vi "fpga_setup.vi"(8 "error in":errorcluster) -> (0 "error out":errorcluster, 3 "Cluster":cluster{"FPGA VI Reference Out":T1})   [LabVIEW 2014]
uses:
  fpga_reference.ctl
  <vilib>/userdefined/High Color/nirio_resource_hc.ctl
  <vilib>/FPGAPlugInAG/PCIe-7842R/niLvFpga_Open_PCIe-7842R.vi
  <vilib>/FPGAPlugInAG/PCIe-7842R/niLvFpga_Reset_PCIe-7842R.vi
  <vilib>/rvi/interface/nirviOpenFPGA/nirviOpenFPGA.xnode
  FPGA Bitfiles/i2cmuxdemux.lvbitx
  <vilib>/rvi/interface/nirviMethod/nirviMethod.xnode
panel:
  # "Open FPGA I2C interface, creating FPGA reference handle, and reset, but don't actually\nstart the hardware yet.  This will stop the hardware if it is already running."
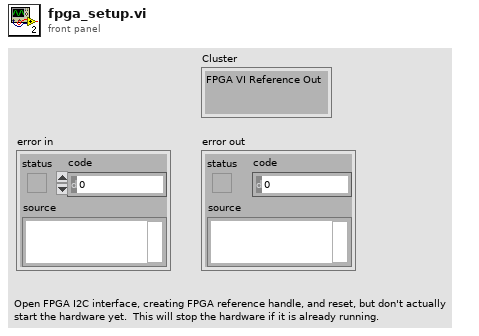
[diagram p1: front panel]
types:
  T1 = typedef "fpga_reference.ctl" = refnum<k20>
  T2 = typedef "nirio_resource_hc.ctl" = tag
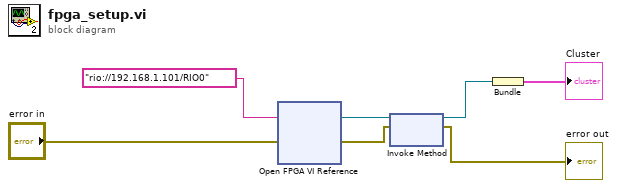
[diagram p0: block diagram]
diagram:
  n1 = xnode "Open FPGA VI Reference"("error in"="error in", "resource name"=T2 "rio://192.168.1.101/RIO0") -> ("FPGA VI Reference Out"=w5:T1, "error out"=w4:errorcluster)
  n2 = xnode "Invoke Method"("FPGA VI Reference In"=w5, "error in"=w4) -> ("FPGA VI Reference Out"=w2:T1, "error out"=→"error out":errorcluster)
  n3 = Bundle("FPGA VI Reference Out"=w2) -> (→"Cluster":cluster{"FPGA VI Reference Out":T1})  [unwired: 1 in]
